vi "ClimbExecute_CtrlOnly.vi"(8 "Left Hard Limit Rev":bool, 9 "Left Sensor Position":dbl, 10 "Right Hard Limit Rev":bool, 11 "Right Sensor Position":dbl) -> (0 "Left Dmd":dbl, 1 "Left Output":dbl, 2 "Right Demand":dbl, 3 "Right Output":dbl, 4 "Left OnTarget":bool, 5 "Right OnTarget":bool)   [LabVIEW 2023]
uses:
  <vilib>/Rock Robotics/WPI/ThirdParty/JAS_Junk/TrajLib/VI/BoolCmd_Recv_Internal.vi
  <vilib>/Rock Robotics/WPI/ThirdParty/JAS_Junk/TrajLib/VI/BoolCmd_ObtainQueue.vi
  <vilib>/Rock Robotics/Network Tables/NT Write Number.vi
  <vilib>/Rock Robotics/Network Tables/NT Write Boolean.vi
  <vilib>/Rock Robotics/WPI/ThirdParty/JAS_Junk/TrajLib/Trajectory_Library.lvlib
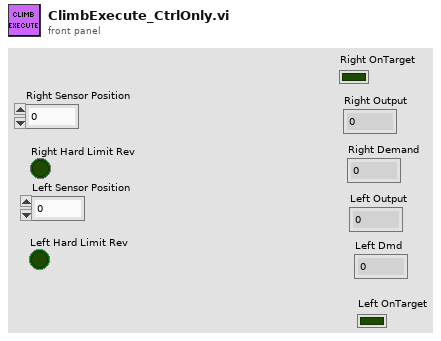
[diagram p1: front panel]
types:
  T1 = typedef "Trajectory_Library.lvlib/PosCtrl_Tuning_Type.ctl" = cluster{"Slope":dbl, "Offset":dbl, "Error Deadband":dbl, "At Reference Count":i32, "Negate Output":bool, "Max Allowd Position":dbl, "Min Allowd Position":dbl}
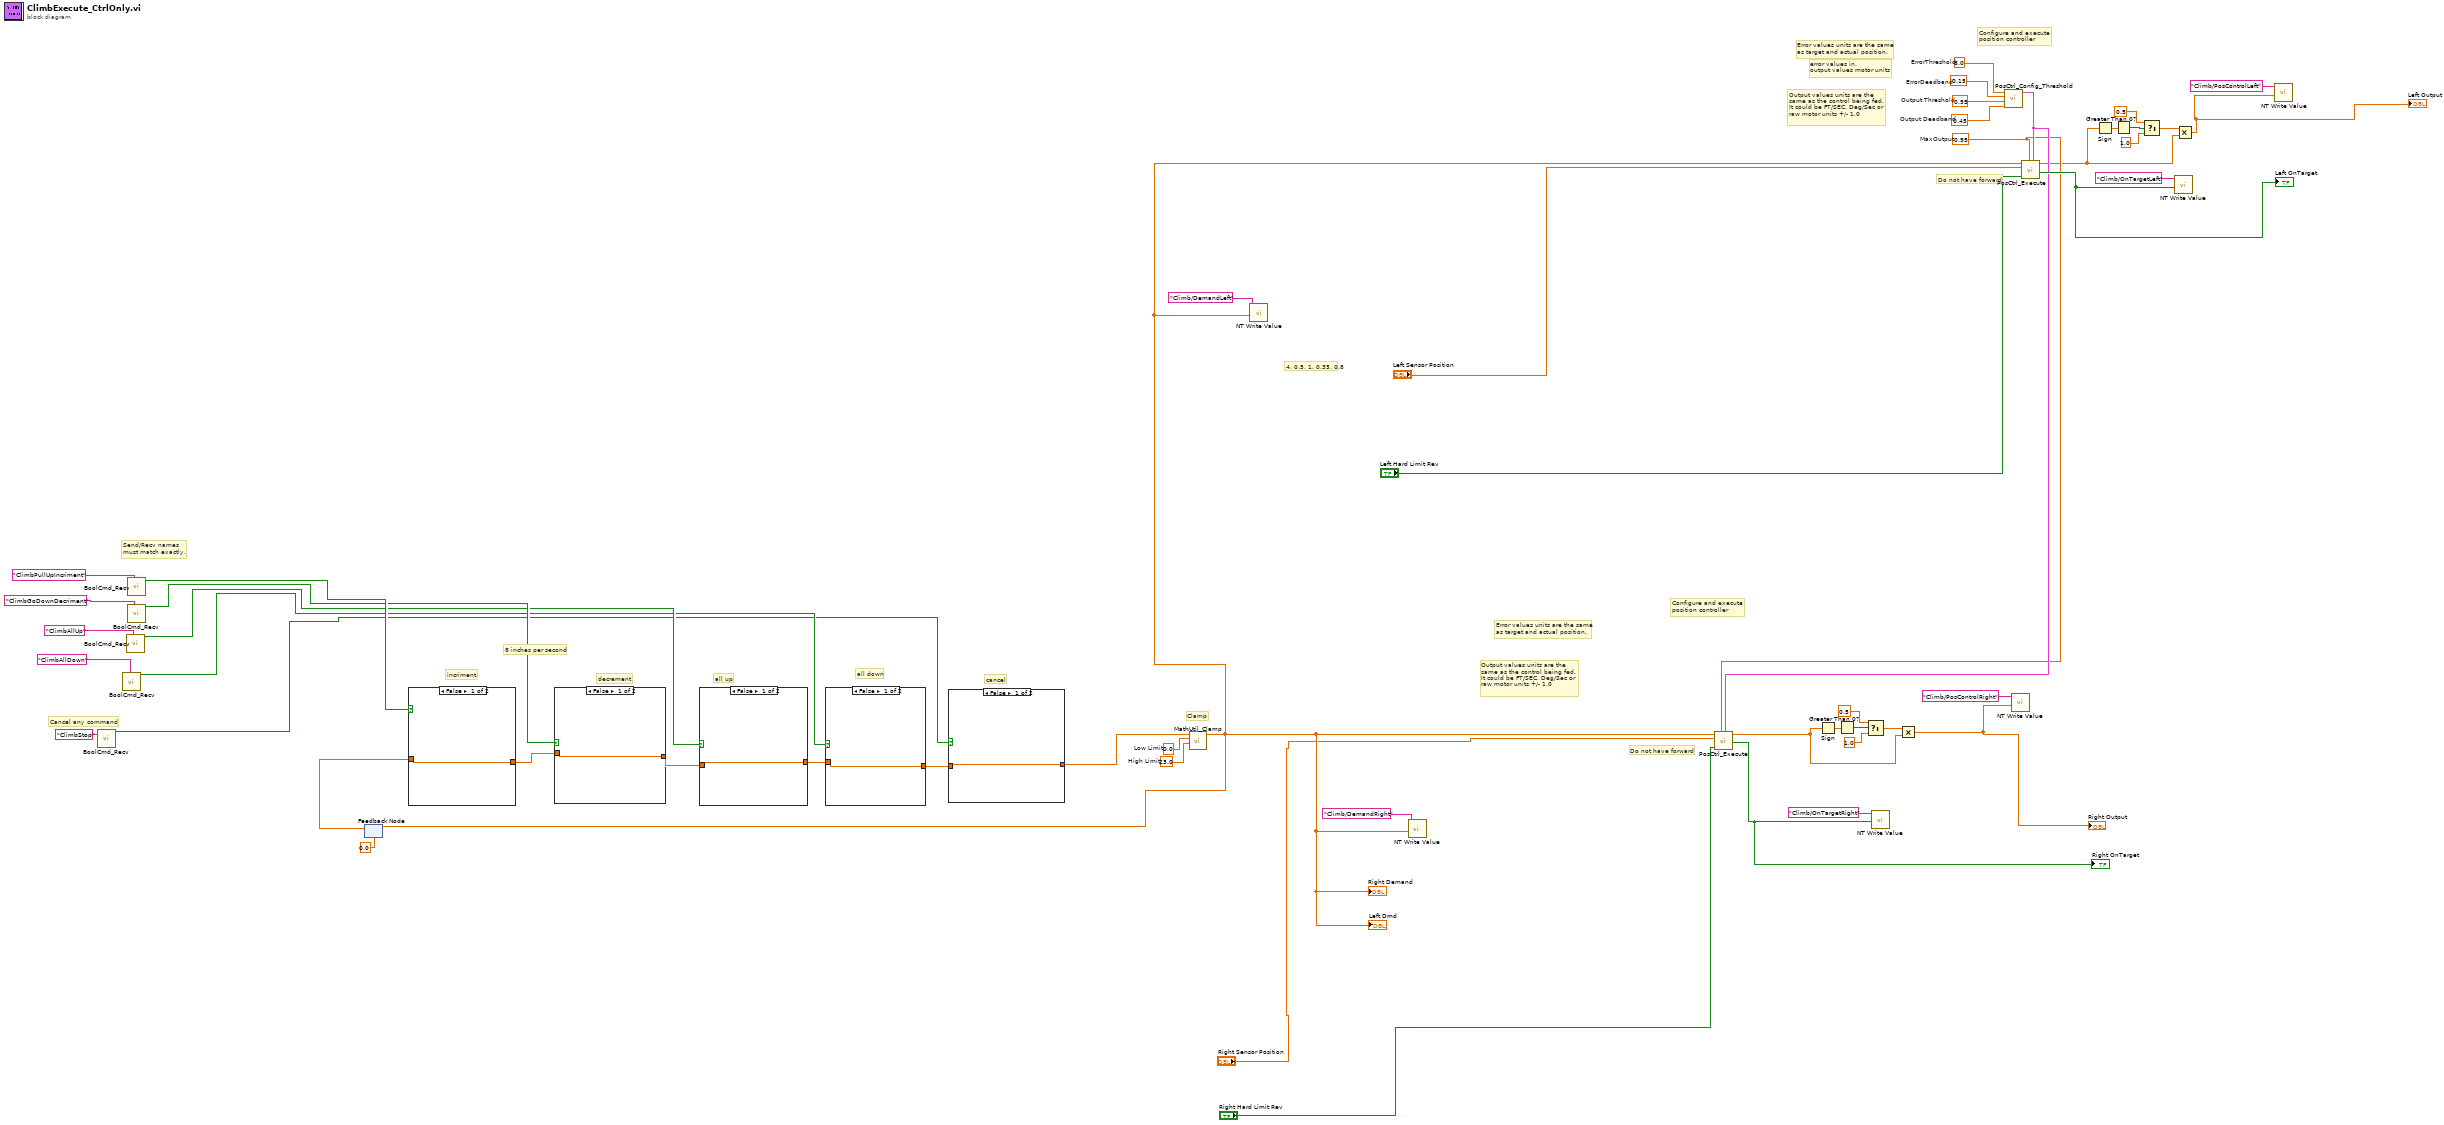
[diagram p0: block diagram]
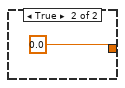
[diagram p3: hidden frame]
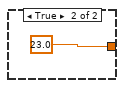
[diagram p4: hidden frame]
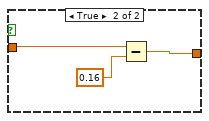
[diagram p5: hidden frame]
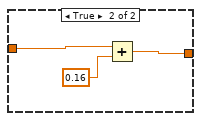
[diagram p6: hidden frame]
diagram:
  w32 = 23.0  # High Limit
  w31 = 0.0  # Low Limit
  w15 = 0.95  # MaxOutput
  w52 = 8.0  # ErrorThreshold
  w51 = 0.15  # ErrorDeadband
  w50 = 0.95  # Output Threshold
  w49 = 0.45  # Output Deadband
  # "cancel"
  # "Clamp"
  # "8 inches per second"
  # "all down"
  # "all up"
  # "decrement"
  # "incriment"
  # "Cancel any command"
  # "Send/Recv names\nmust match exactly."
  # "error values in.\noutput values motor units"
  # "Do not have forward"
  # "Output values units are the\nsame as the control being fed.  \nIt could be FT/SEC, Deg/Sec or\nraw motor units +/- 1.0"
  # "Error values units are the same \nas target and actual position."
  # "Configure and execute \nposition controller"
  # "Do not have forward"
  # "Output values units are the\nsame as the control being fed.  \nIt could be FT/SEC, Deg/Sec or\nraw motor units +/- 1.0"
  # "Error values units are the same \nas target and actual position."
  # "Configure and execute \nposition controller"
  # "4, 0.5, 1, 0.35, 0.8"
  n1 = call <vilib>:"BoolCmd_Recv.vi"("Command Name"="ClimbStop") -> ("New Request"=w17:bool)  [unwired: 9 in, 1 out]
  n2 = call <vilib>:"BoolCmd_Recv.vi"("Command Name"="ClimbAllDown") -> ("New Request"=w18:bool)  [unwired: 9 in, 1 out]
  n3 = call <vilib>:"BoolCmd_Recv.vi"("Command Name"="ClimbAllUp") -> ("New Request"=w19:bool)  [unwired: 9 in, 1 out]
  n4 = call <vilib>:"BoolCmd_Recv.vi"("Command Name"="ClimbPullUpIncriment") -> ("New Request"=w21:bool)  [unwired: 9 in, 1 out]
  n5 = call <vilib>:"BoolCmd_Recv.vi"("Command Name"="ClimbGoDownDecriment") -> ("New Request"=w20:bool)  [unwired: 9 in, 1 out]
  n6 = feedback #1(0.0 ("false")) -> (w36:dbl)
  n7 = case shown="False" w21 {
    tunnel: w36 -> [w53 w56]
    tunnel: [w53 w54] -> w35
    frame False {
    }
    frame True {
      n8 = Add(x=w56, y=0.16) -> (x+y=w54:dbl)
    }
  }
  n9 = case shown="False" w20 {
    tunnel: w35 -> [w57 w59]
    tunnel: [w57 w58] -> w34
    frame False {
    }
    frame True {
      n10 = Subtract(x=w59, y=0.16) -> (x-y=w58:dbl)
    }
  }
  n11 = case shown="False" w19 {
    tunnel: w34 -> [w61 _]
    tunnel: [w61 23.0 ("y")] -> w33
    frame False {
    }
    frame True {
    }
  }
  n12 = case shown="False" w18 {
    tunnel: w33 -> [w63 _]
    tunnel: [w63 0.0 ("y")] -> w30
    frame False {
    }
    frame True {
    }
  }
  n13 = case shown="False" w17 {
    tunnel: w30 -> [w65 w66]
    tunnel: [w65 w66] -> w29
    frame False {
    }
    frame True {
    }
  }
  n14 = call <vilib>:"MathUtil_Clamp.vi"("High Limit"=w32, "Low Limit"=w31, "Value"=w29) -> ("Result"=w26:dbl)  [unwired: 8 in]
  "Left Dmd" <- w26
  "Right Demand" <- w26
  n15 = feedback-in #1(w26) -> ()
  n16 = call-poly <vilib>:"NT Write Value.vi"("value"=w26, "name"="Climb/DemandLeft") -> ()  [unwired: 9 in, 1 out]
  n17 = call-poly <vilib>:"NT Write Value.vi"("value"=w26, "name"="Climb/DemandRight") -> ()  [unwired: 9 in, 1 out]
  n18 = call <vilib>:"PosCtrl_Config_Threshold.vi"("Output Deadband"=w49, "Output Threshold"=w50, "ErrorDeadband"=w51, "ErrorThreshold"=w52) -> ("PosCtrl_Config_Params"=w16:T1)  [unwired: 7 in]
  n19 = call <vilib>:"PosCtrl_Execute.vi"("PosCtrl_Config_Params"=w16, "MaxOutput"=w15, "Rev Limit Switch"="Right Hard Limit Rev", "CurrentPosition"="Right Sensor Position", "TargetPosition"=w26) -> ("OnTarget"=w28:bool, "Output"=w2:dbl)  [unwired: 4 in, 1 out]
  "Right OnTarget" <- w28
  n20 = Sign(1:w2) -> (0:w7:dbl)
  n21 = Greater Than 0?(x=w7) -> (x > 0?=w6:bool)
  n22 = Select(t=0.5, s=w6, f=1.0) -> (s? t:f=w3:dbl)
  n23 = call-poly <vilib>:"NT Write Value.vi"("value"=w28, "name"="Climb/OnTargetRight") -> ()  [unwired: 9 in, 1 out]
  n24 = Multiply(x=w3, y=w2) -> (x*y=w1:dbl)
  "Right Output" <- w1
  n25 = call-poly <vilib>:"NT Write Value.vi"("value"=w1, "name"="Climb/PosControlRight") -> ()  [unwired: 9 in, 1 out]
  n26 = call <vilib>:"PosCtrl_Execute.vi"("PosCtrl_Config_Params"=w16, "MaxOutput"=w15, "Rev Limit Switch"="Left Hard Limit Rev", "CurrentPosition"="Left Sensor Position", "TargetPosition"=w26) -> ("OnTarget"=w27:bool, "Output"=w9:dbl)  [unwired: 4 in, 1 out]
  "Left OnTarget" <- w27
  n27 = Sign(1:w9) -> (0:w14:dbl)
  n28 = Greater Than 0?(x=w14) -> (x > 0?=w13:bool)
  n29 = Select(t=0.5, s=w13, f=1.0) -> (s? t:f=w10:dbl)
  n30 = call-poly <vilib>:"NT Write Value.vi"("value"=w27, "name"="Climb/OnTargetLeft") -> ()  [unwired: 9 in, 1 out]
  n31 = Multiply(x=w10, y=w9) -> (x*y=w8:dbl)
  "Left Output" <- w8
  n32 = call-poly <vilib>:"NT Write Value.vi"("value"=w8, "name"="Climb/PosControlLeft") -> ()  [unwired: 9 in, 1 out]
